vi "plus and minus.vi"(9 "b":i32, 10 "a":i32) -> (1 "a-b":i32, 2 "a+b":i32)   [LabVIEW 2013]
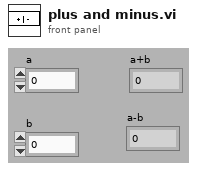
[diagram p1: front panel]
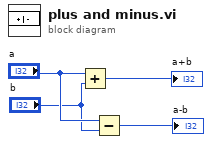
[diagram p0: block diagram]
diagram:
  n1 = Add(x="a", y="b") -> (x+y=→"a+b":i32)
  n2 = Subtract(x="a", y="b") -> (x-y=→"a-b":i32)
